vi "plot_main.vi"(10 "Break":refnum<vi>) -> ()   [LabVIEW 2019]
uses:
  controls/open_picButton.ctl
  controls/hydrolyse_picButton.ctl
  controls/methane_picButton.ctl
  controls/storage_picButton.ctl
  lib/libSimulationControl/libSimulationControl.lvlib
panel:
  in  "WindowTitle":string
  out "Load cluster":T1
  in  "Load Storage":T2 caption="Load Simulation"
  in  "Load Methane":T3 caption="Load Simulation"
  in  "Load Hydrolysis":T4 caption="Load Simulation"
  out "Output File Loaded?":bool
  in  "Close":bool
  out "# Lines Plot":i32
  in  "Parameters to Plot":string(tree)="_3"
  out "Output Files Path":path caption="selected path"
  in  "Load File":T5
  in  "Clear Plot Selection":bool
  in  "Plot":bool
  # "Biogas Plotter"
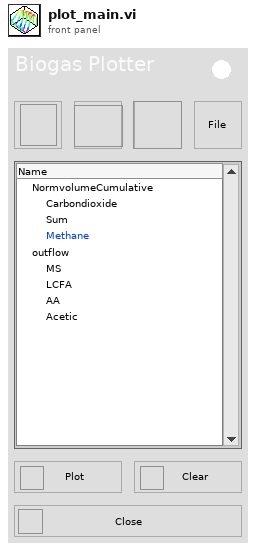
[diagram p1: front panel]
types:
  T1 = cluster{"# Lines Plot":refnum<vi>, "Output File Loaded?":refnum<vi>, "Parameters to Plot":refnum<vi>, "Output Files Path":refnum<vi>}
  T2 = typedef "storage_picButton.ctl" = bool
  T3 = typedef "methane_picButton.ctl" = bool
  T4 = typedef "hydrolyse_picButton.ctl" = bool
  T5 = typedef "open_picButton.ctl" = bool
  T6 = typedef "LVPoint32TypeDef.ctl" = cluster{"Horizontal":i32, "Vertical":i32}
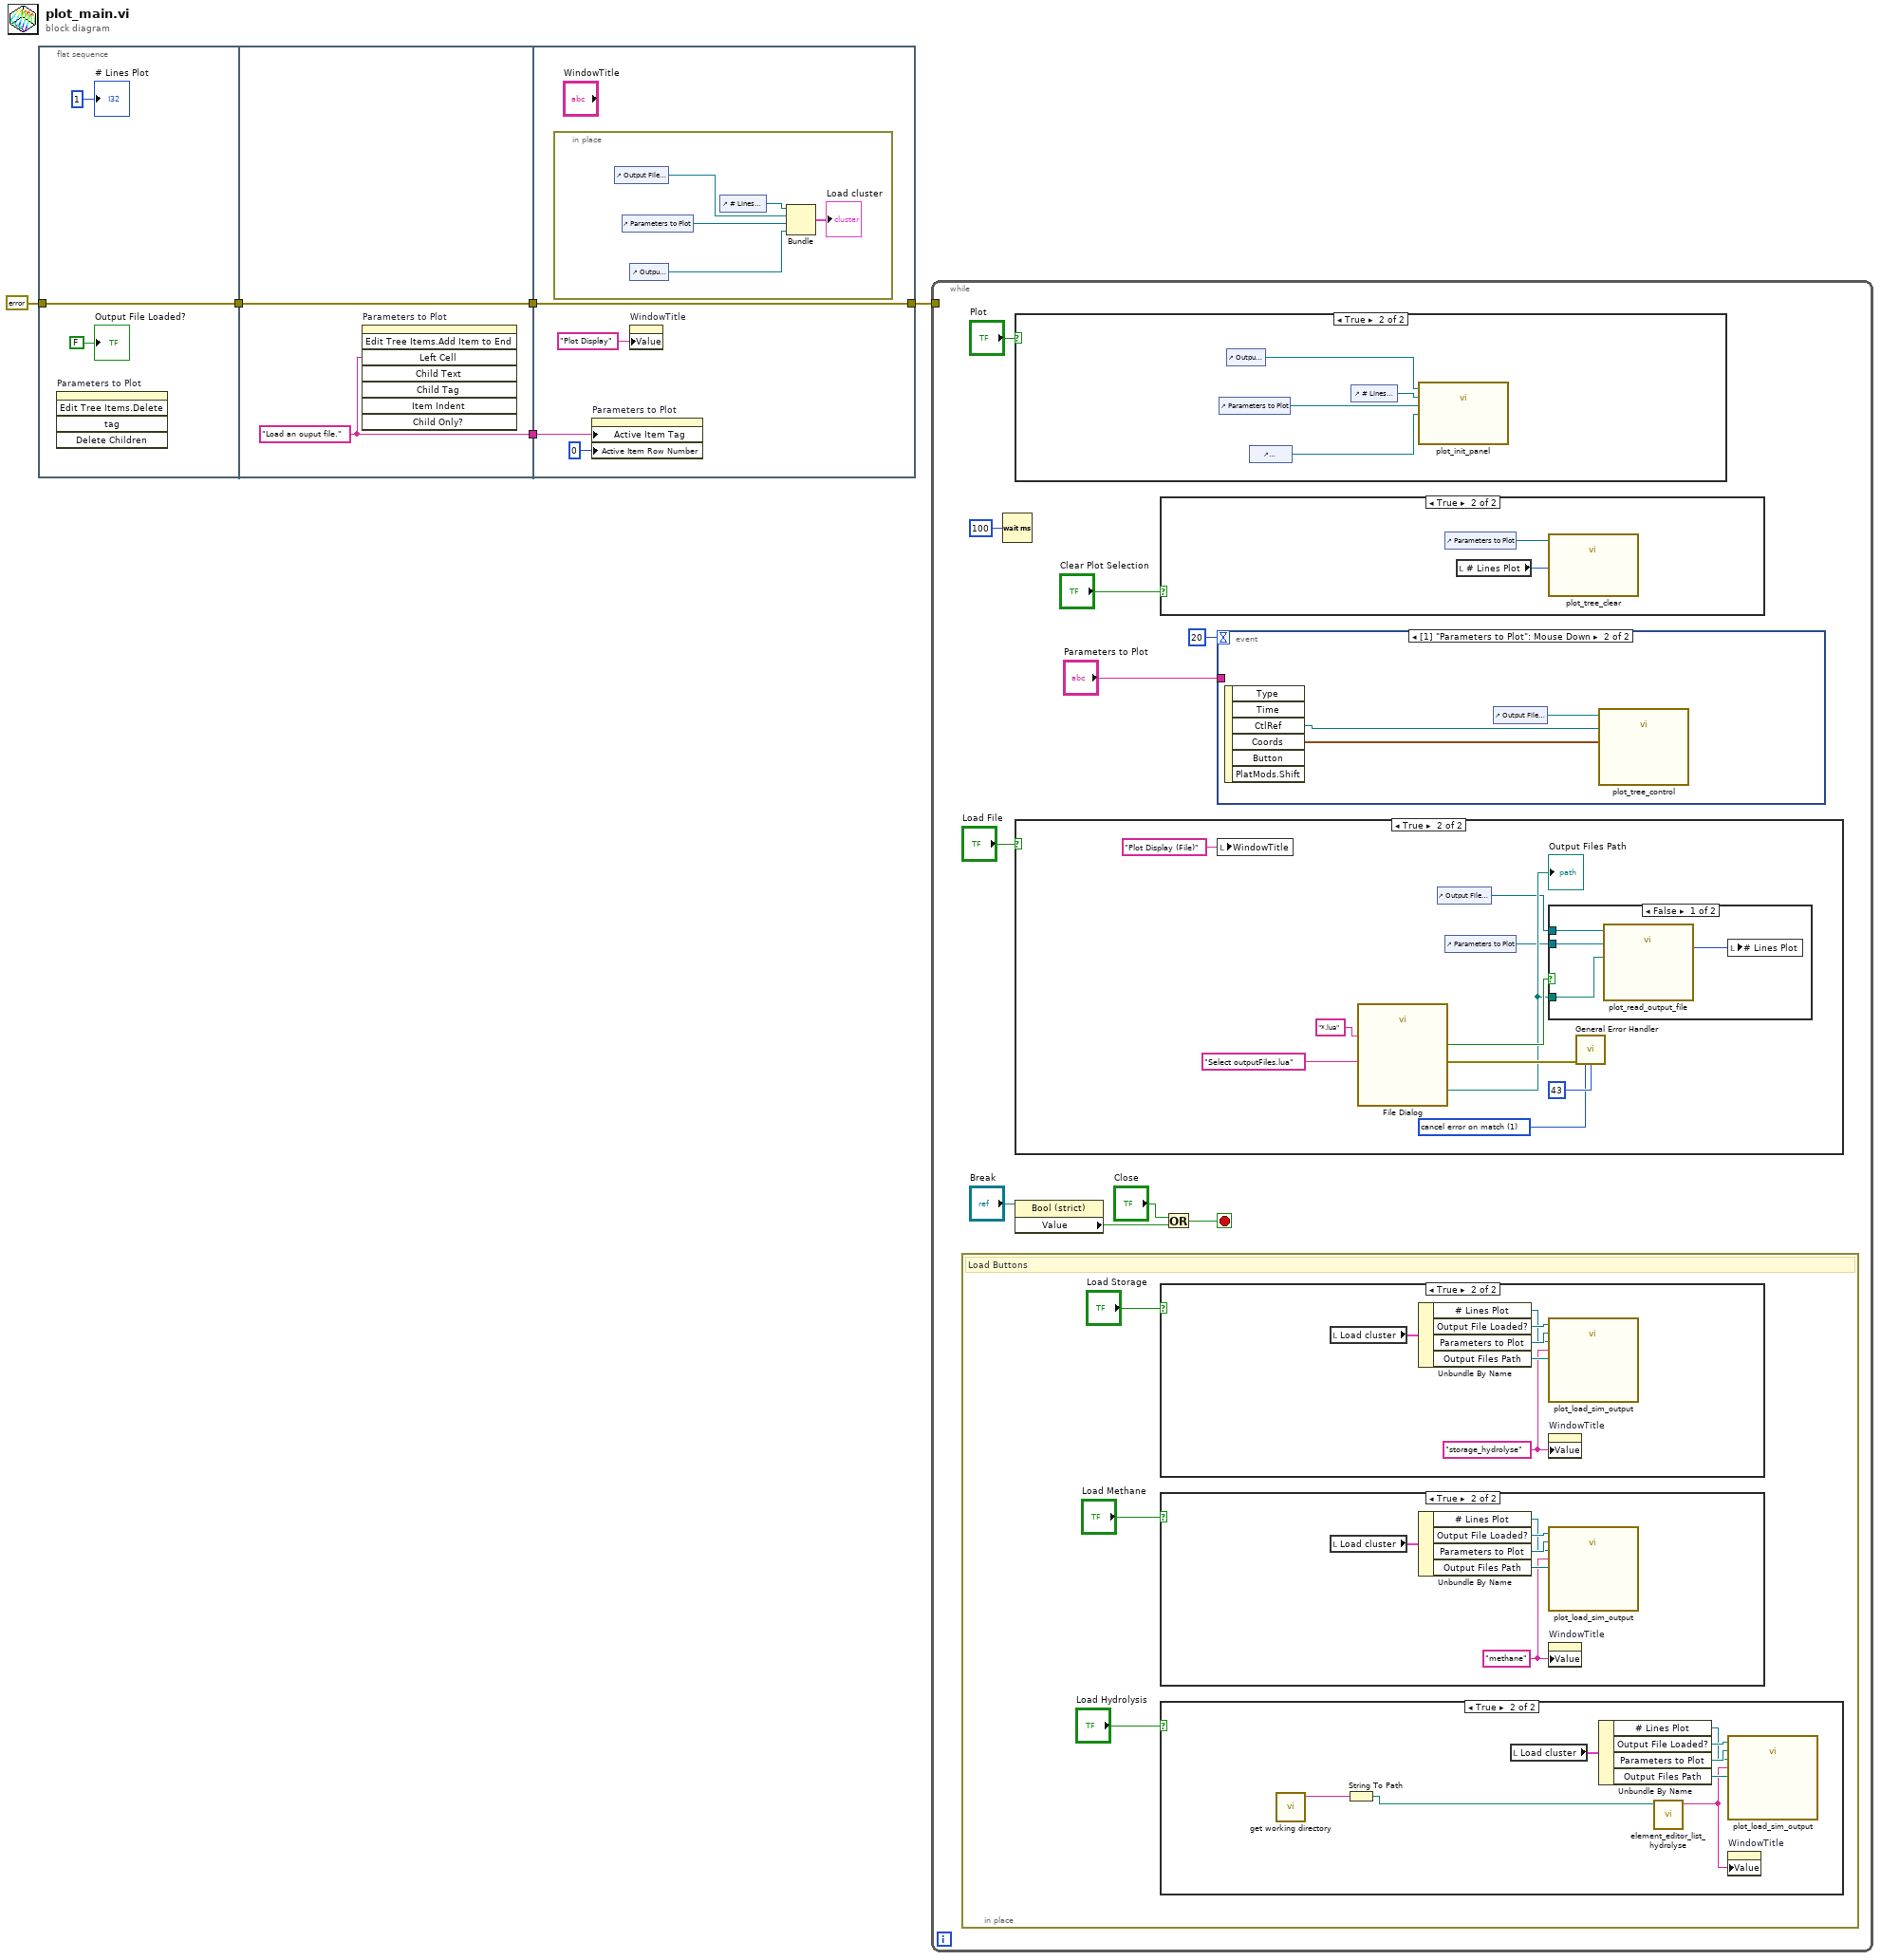
[diagram p0: block diagram]
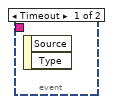
[diagram p8: hidden frame]
diagram:
  n1 = flat-sequence {
    tunnel: [w6] -> w3
    tunnel: errorcluster {"status"=FALSE, "code"=0, "source"=""} ("error constant") -> [w6]
    tunnel: [w10] -> w5
    tunnel: w3 -> [w9]
    tunnel: [w9] -> w2
    tunnel: w5 -> [w14]
    tunnel: w2 -> [w12]
    tunnel: [w12] -> w1
    frame #0 {
      n2 = invoke on="Parameters to Plot" class="Tree (strict)" method="Edit Tree Items.Delete"() -> ()  [unwired: 5 in, 5 out]
      "Output File Loaded?" <- FALSE ("Output File Loaded?")
      "# Lines Plot" <- 1 ("# Lines Plot")
    }
    frame #1 {
      w10 = "Load an ouput file." ("Left Cell String")
      n3 = invoke on="Parameters to Plot" class="Tree (strict)" method="Edit Tree Items.Add Item to End"("Left Cell"=w10) -> ()  [unwired: 7 in, 8 out]
    }
    frame #2 {
      n4 = in-place {
        n5 = control-ref of="Output File Loaded?"() -> (w18:refnum<vi>)
        n6 = control-ref of="Parameters to Plot"() -> (w17:refnum<vi>)
        n7 = control-ref of="Output Files Path"() -> (w16:refnum<vi>)
        n8 = control-ref of="# Lines Plot"() -> (w19:refnum<vi>)
        n9 = Bundle("# Lines Plot"=w19, "Output File Loaded?"=w18, "Parameters to Plot"=w17, "Output Files Path"=w16) -> (→"Load cluster":T1)  [unwired: 1 in]
      }
      n10 = property on="Parameters to Plot" class="Tree (strict)"("Active Item Tag"=w14, "Active Item Row Number"=0 ("Active Item:Row Number")) -> ()  [unwired: 2 in, 2 out]
      n11 = property on="WindowTitle" class="Str"("Value"="Plot Display" ("WindowTitle")) -> ()  [unwired: 2 in, 2 out]
    }
  }
  n12 = while {
    tunnel: w1 -> [_]
    stop <- w21 stop-if-true
    n13 = in-place {
      # "Load Buttons"
      n14 = case shown="True" "Load Storage" {
        frame False {
        }
        frame True {
          w33 = "storage_hydrolyse" ("Folder")
          n15 = local read "Load cluster"() -> (w38:T1)
          n16 = Unbundle By Name(w38) -> ("# Lines Plot"=w35:refnum<vi>, "Output File Loaded?"=w37:refnum<vi>, "Parameters to Plot"=w36:refnum<vi>, "Output Files Path"=w34:refnum<vi>)
          n17 = call "plot_load_sim_output.vi"("Output Files Path"=w34, "Folder"=w33, "# Lines Plot"=w35, "Parameters to Plot"=w36, "Output File Loaded?"=w37) -> ()  [unwired: 7 in]
          n18 = property on="WindowTitle" class="Str"("Value"=w33) -> ()  [unwired: 2 in, 2 out]
        }
      }
      n19 = case shown="True" "Load Methane" {
        frame False {
        }
        frame True {
          w47 = "methane" ("Folder")
          n20 = local read "Load cluster"() -> (w52:T1)
          n21 = Unbundle By Name(w52) -> ("# Lines Plot"=w49:refnum<vi>, "Output File Loaded?"=w51:refnum<vi>, "Parameters to Plot"=w50:refnum<vi>, "Output Files Path"=w48:refnum<vi>)
          n22 = call "plot_load_sim_output.vi"("Output Files Path"=w48, "Folder"=w47, "# Lines Plot"=w49, "Parameters to Plot"=w50, "Output File Loaded?"=w51) -> ()  [unwired: 7 in]
          n23 = property on="WindowTitle" class="Str"("Value"=w47) -> ()  [unwired: 2 in, 2 out]
        }
      }
      n24 = case shown="True" "Load Hydrolysis" {
        frame False {
        }
        frame True {
          n25 = call "get working directory.vi"() -> ("function return"=w41:string)  [unwired: 10 in, 1 out]
          n26 = String To Path(string=w41) -> (path=w39:path)
          n27 = local read "Load cluster"() -> (w46:T1)
          n28 = Unbundle By Name(w46) -> ("# Lines Plot"=w43:refnum<vi>, "Output File Loaded?"=w45:refnum<vi>, "Parameters to Plot"=w44:refnum<vi>, "Output Files Path"=w42:refnum<vi>)
          n29 = call "element_editor_list_hydrolyse.vi"("path"=w39) -> ("Value"=w40:string)  [unwired: 7 in, 3 out]
          n30 = call "plot_load_sim_output.vi"("Output Files Path"=w42, "Folder"=w40, "# Lines Plot"=w43, "Parameters to Plot"=w44, "Output File Loaded?"=w45) -> ()  [unwired: 7 in]
          n31 = property on="WindowTitle" class="Str"("Value"=w40) -> ()  [unwired: 2 in, 2 out]
        }
      }
    }
    n32 = Wait (ms)(milliseconds to wait=u32 100) -> ()  [unwired: 1 out]
    n33 = case shown="True" "Plot" {
      frame False {
      }
      frame True {
        n34 = control-ref of="Parameters to Plot"() -> (w54:refnum<vi>)
        n35 = control-ref of="Output Files Path"() -> (w56:refnum<vi>)
        n36 = control-ref of="WindowTitle"() -> (w53:refnum<vi>)
        n37 = control-ref of="# Lines Plot"() -> (w55:refnum<vi>)
        n38 = call "plot_init_panel.vi"("Window Title"=w53, "Plot Tree"=w54, "#Lines Plot"=w55, "Output Files Path"=w56) -> ()  [unwired: 8 in]
      }
    }
    n39 = case shown="True" "Load File" {
      frame False {
      }
      frame True {
        w64 = 1 items=["no exception", "cancel error on match", "set error on match"] ("[exception action] (none:0)")
        n40 = local write "WindowTitle"("Plot Display (File)" ("WindowTitle")) -> ()
        n41 = call "File Dialog"("prompt"="Select outputFiles.lua", "pattern (all files)"="*.lua") -> ("selected path"=w62:path, "cancelled"=w63:bool, "error out"=w66:errorcluster)  [unwired: 10 in, 1 out]
        "Output Files Path" <- w62
        n42 = control-ref of="Output File Loaded?"() -> (w60:refnum<vi>)
        n43 = control-ref of="Parameters to Plot"() -> (w61:refnum<vi>)
        n44 = case shown="False" w63 {
          tunnel: w62 -> [w70 _]
          tunnel: w61 -> [w69 _]
          tunnel: w60 -> [w68 _]
          frame False {
            n45 = call "plot_read_output_file.vi"("TMP Filepath"=w70, "Plot Tree"=w69, "Output File Loaded?"=w68) -> ("# Lines Plot"=w67:i32)  [unwired: 8 in]
            n46 = local write "# Lines Plot"(w67) -> ()
          }
          frame True {
          }
        }
        n47 = call <vilib>:"General Error Handler.vi"("error in (no error)"=w66, "[exception action] (none:0)"=w64, "[exception code]"=43) -> ()  [unwired: 8 in, 5 out]
      }
    }
    n48 = property class="Bool (strict)"(reference="Break") -> ("Value"=w22:bool)  [unwired: 1 in, 2 out]
    n49 = case shown="True" "Clear Plot Selection" {
      frame False {
      }
      frame True {
        n50 = control-ref of="Parameters to Plot"() -> (w74:refnum<vi>)
        n51 = local read "# Lines Plot"() -> (w75:i32)
        n52 = call "plot_tree_clear.vi"("# Lines Plot"=w75, "Plot Tree"=w74) -> ()  [unwired: 10 in]
      }
    }
    n53 = Or(x="Close", y=w22) -> (x .or. y?=w21:bool)
    n54 = event shown="[1] \"Parameters to Plot\": Mouse Down" {
      selector: _ -> [_ _]
      dyn-events: _ -> [_ _]
      timeout: 20 -> [_ _]
      tunnel: "Parameters to Plot" -> [_ _]
      event Timeout {
        n55 = event-data() -> ()  [unwired: 1 in, 2 out]
      }
      event "Parameters to Plot": Mouse Down {
        n56 = event-data() -> ("CtlRef"=w73:refnum<vi>, "Coords"=w72:T6)  [unwired: 1 in, 4 out]
        n57 = control-ref of="Output File Loaded?"() -> (w71:refnum<vi>)
        n58 = call "plot_tree_control.vi"("Point"=w72, "Plot Tree"=w73, "Output File Loaded?"=w71) -> ()  [unwired: 9 in]
      }
    }
  }
